vi "Compiled.Get Sim DTCs.vi"(8 "error in (no error)":errorcluster, 10 "Node Ref in":T1 format="%.0x", 11 "Addon Ref in":T1 format="%.0x") -> (0 "error out":errorcluster, 1 "Sim DTCs":T2 {"DM1.Ref"."Data Reference" format="%.0x"; "DM1.Enable.Ref"."Data Reference" format="%.0x"; "DM2.Ref"."Data Reference" format="%.0x"; "DM2.Enable.Ref"."Data Reference" format="%.0x"}, 2 "Node Ref out":T1 format="%.0x", 3 "Addon Ref out":T1=18446744073709551615 format="%.0x")   [LabVIEW 2019, in "J1939 Addon System Explorer.lvlib"]
uses:
  J1939 Addon System Explorer.lvlib
  Addon Shared/Types/Compiled Simulated Settings.ctl
  <vilib>/NI VeriStand/Custom Device API/Block Data Reference.ctl
  <vilib>/NI VeriStand/Custom Device API/Data Reference.ctl
  <vilib>/NI VeriStand/Custom Device API/Custom Device Item Ref.ctl
  <vilib>/NI VeriStand/Custom Device API/Data Access Type.ctl
  Addon Shared/SubVIs/Constants.vi
  Addon Shared/J1939 Addon Shared.lvlib
  <vilib>/NI VeriStand/Custom Device API/Custom Device API.lvlib
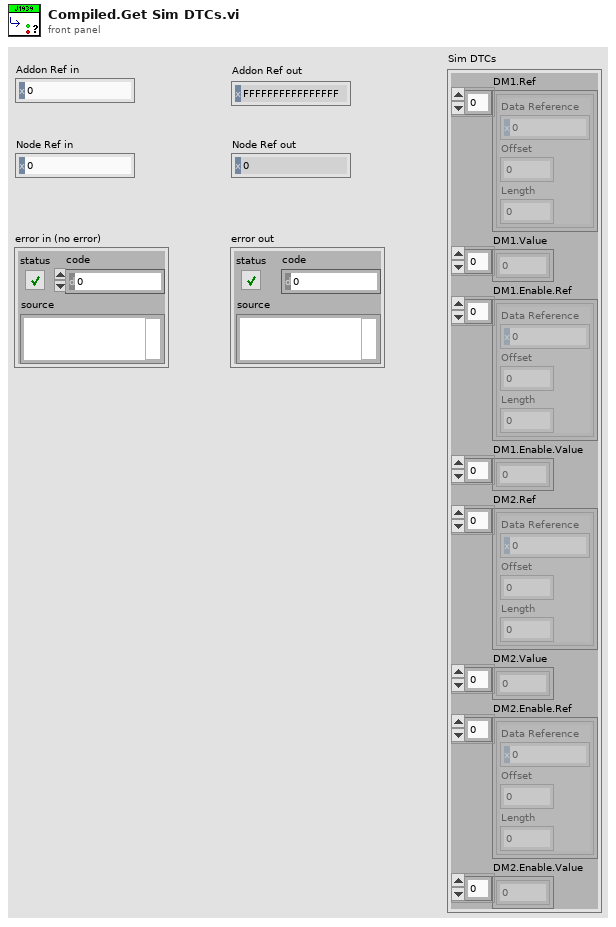
[diagram p1: front panel]
types:
  T1 = typedef "Custom Device API.lvlib/Custom Device Item Ref.ctl" = u64
  T2 = typedef "J1939 Addon Shared.lvlib/Compiled Simulated Settings.ctl" = cluster{"DM1.Ref":T3[], "DM1.Value":dbl[], "DM1.Enable.Ref":T3[], "DM1.Enable.Value":dbl[], "DM2.Ref":T3[], "DM2.Value":dbl[], "DM2.Enable.Ref":T3[], "DM2.Enable.Value":dbl[]}
  T3 = typedef "Custom Device API.lvlib/Block Data Reference.ctl" = cluster{"Data Reference":T4, "Offset":u64, "Length":u64}
  T4 = typedef "Custom Device API.lvlib/Data Reference.ctl" = i32
  T5 = typedef "Custom Device API.lvlib/Data Access Type.ctl" = enum16{"Read", "Write"}
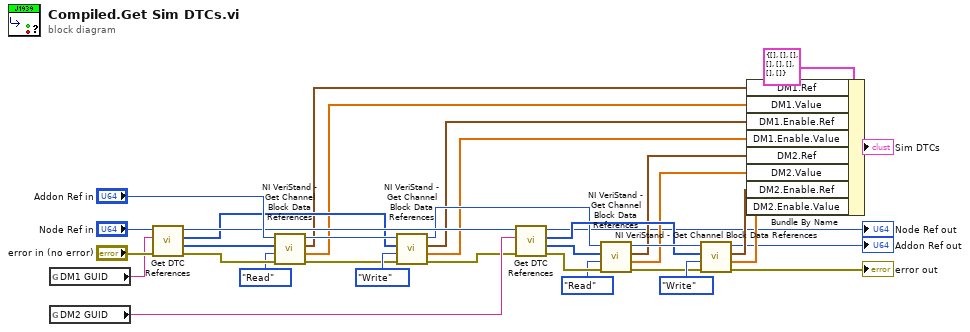
[diagram p0: block diagram]
diagram:
  n1 = global read "Constants.vi" "DM1 GUID"() -> (w30:string)
  n2 = global read "Constants.vi" "DM2 GUID"() -> (w29:string)
  n3 = call "Get DTC References.vi"("error in (no error)"="error in (no error)", "DM GUID"=w30, "Item Ref in"="Node Ref in") -> ("error out"=w27:errorcluster, "Data"=w26:T1[], "Active"=w12:T1[], "Section Ref out"=w28:T1)  [unwired: 5 in]
  n4 = call <vilib>:"NI VeriStand - Get Channel Block Data References.vi"("error in (no error)"=w27, "Access"=Data_Access_Type."Read", "Channel Refs"=w26, "Device Ref in"="Addon Ref in") -> ("error out"=w16:errorcluster, "Values Array"=w10:dbl[], "Block Data Refs"=w11:T3[], "Device Ref out"=w14:T1)  [unwired: 4 in]
  n5 = call <vilib>:"NI VeriStand - Get Channel Block Data References.vi"("error in (no error)"=w16, "Access"=Data_Access_Type."Write", "Channel Refs"=w12, "Device Ref in"=w14) -> ("error out"=w15:errorcluster, "Values Array"=w5:dbl[], "Block Data Refs"=w4:T3[], "Device Ref out"=w13:T1)  [unwired: 4 in]
  n6 = call "Get DTC References.vi"("error in (no error)"=w15, "DM GUID"=w29, "Item Ref in"=w28) -> ("error out"=w25:errorcluster, "Data"=w24:T1[], "Active"=w18:T1[], "Section Ref out"=→"Node Ref out":T1)  [unwired: 5 in]
  n7 = call <vilib>:"NI VeriStand - Get Channel Block Data References.vi"("error in (no error)"=w25, "Access"=Data_Access_Type."Read", "Channel Refs"=w24, "Device Ref in"=w13) -> ("error out"=w20:errorcluster, "Values Array"=w7:dbl[], "Block Data Refs"=w6:T3[], "Device Ref out"=w19:T1)  [unwired: 4 in]
  n8 = call <vilib>:"NI VeriStand - Get Channel Block Data References.vi"("error in (no error)"=w20, "Access"=Data_Access_Type."Write", "Channel Refs"=w18, "Device Ref in"=w19) -> ("error out"=→"error out":errorcluster, "Values Array"=w9:dbl[], "Block Data Refs"=w8:T3[], "Device Ref out"=→"Addon Ref out":T1)  [unwired: 4 in]
  n9 = Bundle By Name(cluster=T2 {"DM1.Ref"=[], "DM1.Value"=[], "DM1.Enable.Ref"=[], "DM1.Enable.Value"=[], "DM2.Ref"=[], "DM2.Value"=[], "DM2.Enable.Ref"=[], "DM2.Enable.Value"=[]} ("Sim DTCs"), "DM1.Ref"=w11, "DM1.Value"=w10, "DM1.Enable.Ref"=w4, "DM1.Enable.Value"=w5, "DM2.Ref"=w6, "DM2.Value"=w7, "DM2.Enable.Ref"=w8, "DM2.Enable.Value"=w9) -> (→"Sim DTCs":T2)
